vi "DPT RMC Check Range.vi"(4 "Complete":T1, 6 "In Range?":bool, 8 "Error In":errorcluster) -> (0 "Error Out":errorcluster, 3 "End":bool)   [LabVIEW 2016, in "File Setup.lvlib"]
uses:
  File Setup.lvlib
  Custom Pallet Controls/Custom Pallet Forward.ctl
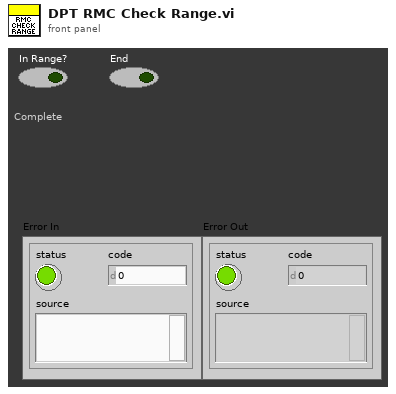
[diagram p1: front panel]
types:
  T1 = typedef "Custom Pallet Forward.ctl" = bool
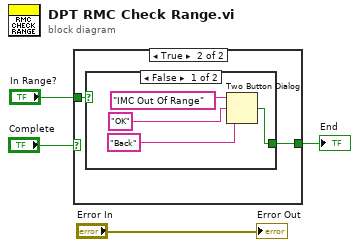
[diagram p0: block diagram]
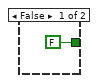
[diagram p2: hidden frame]
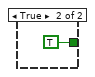
[diagram p3: hidden frame]
diagram:
  n1 = case shown="True" "Complete" {
    tunnel: "In Range?" -> [_ w7]
    tunnel: [FALSE w6] -> w3
    frame False {
    }
    frame True {
      n2 = case shown="False" w7 {
        tunnel: [w8 TRUE] -> w6
        frame False {
          n3 = Two Button Dialog(message="IMC Out Of Range", 1:"Back" ("F button name (\"Cancel\")"), 2:"OK" ("T button name (\"OK\")")) -> (T button?=w8:bool)
        }
        frame True {
        }
      }
    }
  }
  "End" <- w3
  "Error Out" <- "Error In"
